vi "Dynamic Launch Nested Actor.vi"(8 "error in (no error)":errorcluster, 11 "UI ActorTop in":refnum<class "UI_Up_Down.lvclass">) -> (0 "error out":errorcluster, 3 "UI ActorTop out":refnum<class "UI_Up_Down.lvclass">)   [LabVIEW 2021, in "UI_Up_Down.lvclass"]
doc: "Use Launch Nested Actor.vi to dynamic load child VI.\n2015-04-02 12:54:56\n蒋松\njiangsong@outlook.com"
uses:
  UI_Up_Down.lvclass
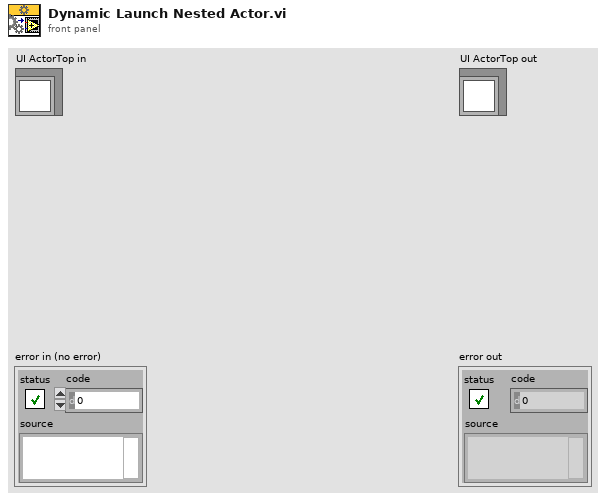
[diagram p1: front panel]
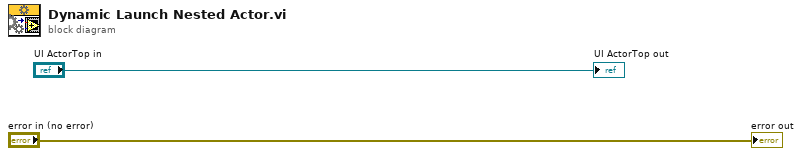
[diagram p0: block diagram]
diagram:
  "error out" <- "error in (no error)"
  "UI ActorTop out" <- "UI ActorTop in"
